vi "Message to Message Option.vi"(11 "Message":string) -> (3 "Message Option":string)   [LabVIEW 2017, in "Git-LabVIEW.lvlib" / "Git Implementation.lvclass"]
uses:
  Git Implementation.lvclass
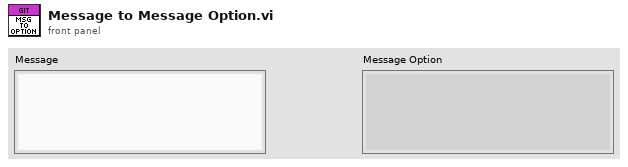
[diagram p1: front panel]
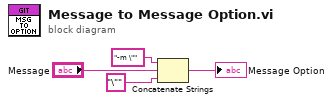
[diagram p0: block diagram]
diagram:
  n1 = Concatenate Strings("-m \"" ("string"), "Message", "\"" ("string")) -> (→"Message Option":string)
